vi "AddAxis.vi"(6 "Units":string, 8 "error in (no error)":errorcluster, 9 "Encoder Resolution":string, 10 "Axis Letter":string, 11 "Controller in":refnum<class "Controller.lvclass">) -> (0 "error out":errorcluster, 3 "Controller out":refnum<class "Controller.lvclass">)   [LabVIEW 2019, in "Controller.lvclass"]
uses:
  Controller.lvclass
  Axis/Axis.lvclass
  Controller.lvclass/Controller.ctl
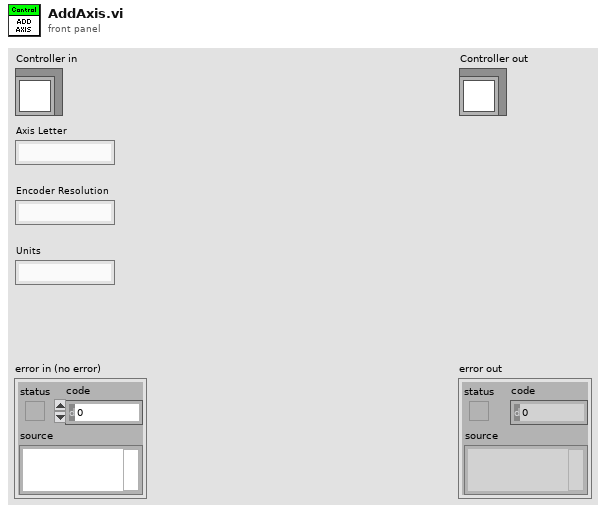
[diagram p1: front panel]
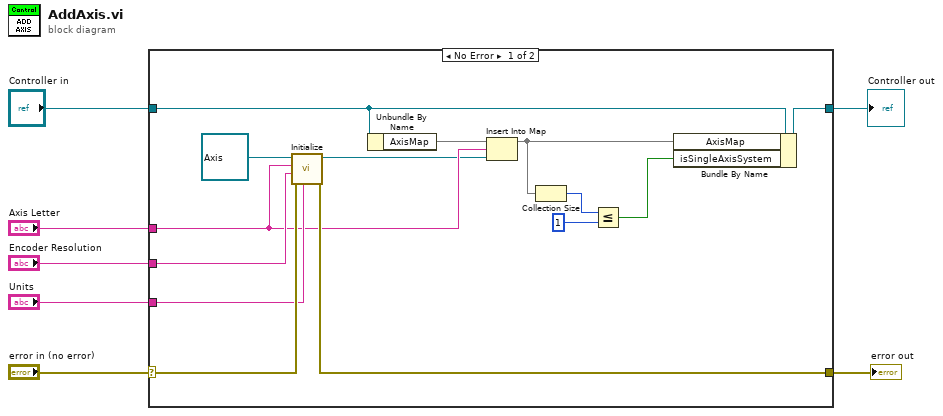
[diagram p0: block diagram]
diagram:
  n1 = case shown="No Error" "error in (no error)" {
    selector: "error in (no error)" -> [w19 w23]
    tunnel: [w18 w23] -> w6
    tunnel: [w16 w22] -> w4
    tunnel: "Controller in" -> [w20 w22]
    tunnel: "Units" -> [w15 _]
    tunnel: "Encoder Resolution" -> [w14 _]
    tunnel: "Axis Letter" -> [w13 _]
    frame No Error {
      n2 = call-dynamic "Initialize.vi"("Current Units"=w15, "error in (no error)"=w19, "Encoder Resolution"=w14, "Axis Letter"=w13, "Axis in"=refnum<class "Axis.lvclass"> refnum ("Axis.lvclass")) -> ("error out"=w18:errorcluster, "Axis out"=w12:refnum<class "Axis.lvclass">)  [unwired: 5 in]
      n3 = Unbundle By Name(w20) -> ("AxisMap"=w17:map{string, refnum<class "Axis.lvclass">})
      n4 = Insert Into Map(map in=w17, key=w13, value=w12) -> (map out=w11:map{string, refnum<class "Axis.lvclass">})  [unwired: 2 out]
      n5 = Collection Size(1:w11) -> (0:w10:i32)
      n6 = Less Or Equal?(x=w10, y=1) -> (x <= y?=w8:bool)
      n7 = Bundle By Name(cluster=w20, "AxisMap"=w11, "isSingleAxisSystem"=w8) -> (w16:refnum<class "Controller.lvclass">)
    }
    frame Error {
    }
  }
  "error out" <- w6
  "Controller out" <- w4
